vi "START6LED.vi"() -> ()   [LabVIEW 2024]
uses:
  <vilib>/Utility/file.llb/Read Delimited Spreadsheet (DBL).vi
panel:
  in  "Flow Rate Lower Limit 2":dbl
  in  "Flow Rate Upper Limit 2":dbl
  in  "Desired Flow Rate 3":dbl format="%_2f"
  in  "Initial RPM  3":dbl format="%_4f"
  in  "stop 2":bool
  out "Boolean":bool
  out "Waveform Chart 3":dbl[](graph)
  out "Waveform Chart 2":dbl[](graph)
  out "Flow Rate":dbl[](graph)
  in  "Color Box":u32(colorbox)
  # "Blood Flow Rate"
  # "Initial LVAD Speed (RPM)"
  # "Desired Flow Rate (L/min)"
  # "LVAD Speed"
  # "Upper Flow Rate Limit (L/min)"
  # "Lower Flow Rate Limit (L/min)"
  # "Optimal Flow State"
  # "Right Heart Waveform"
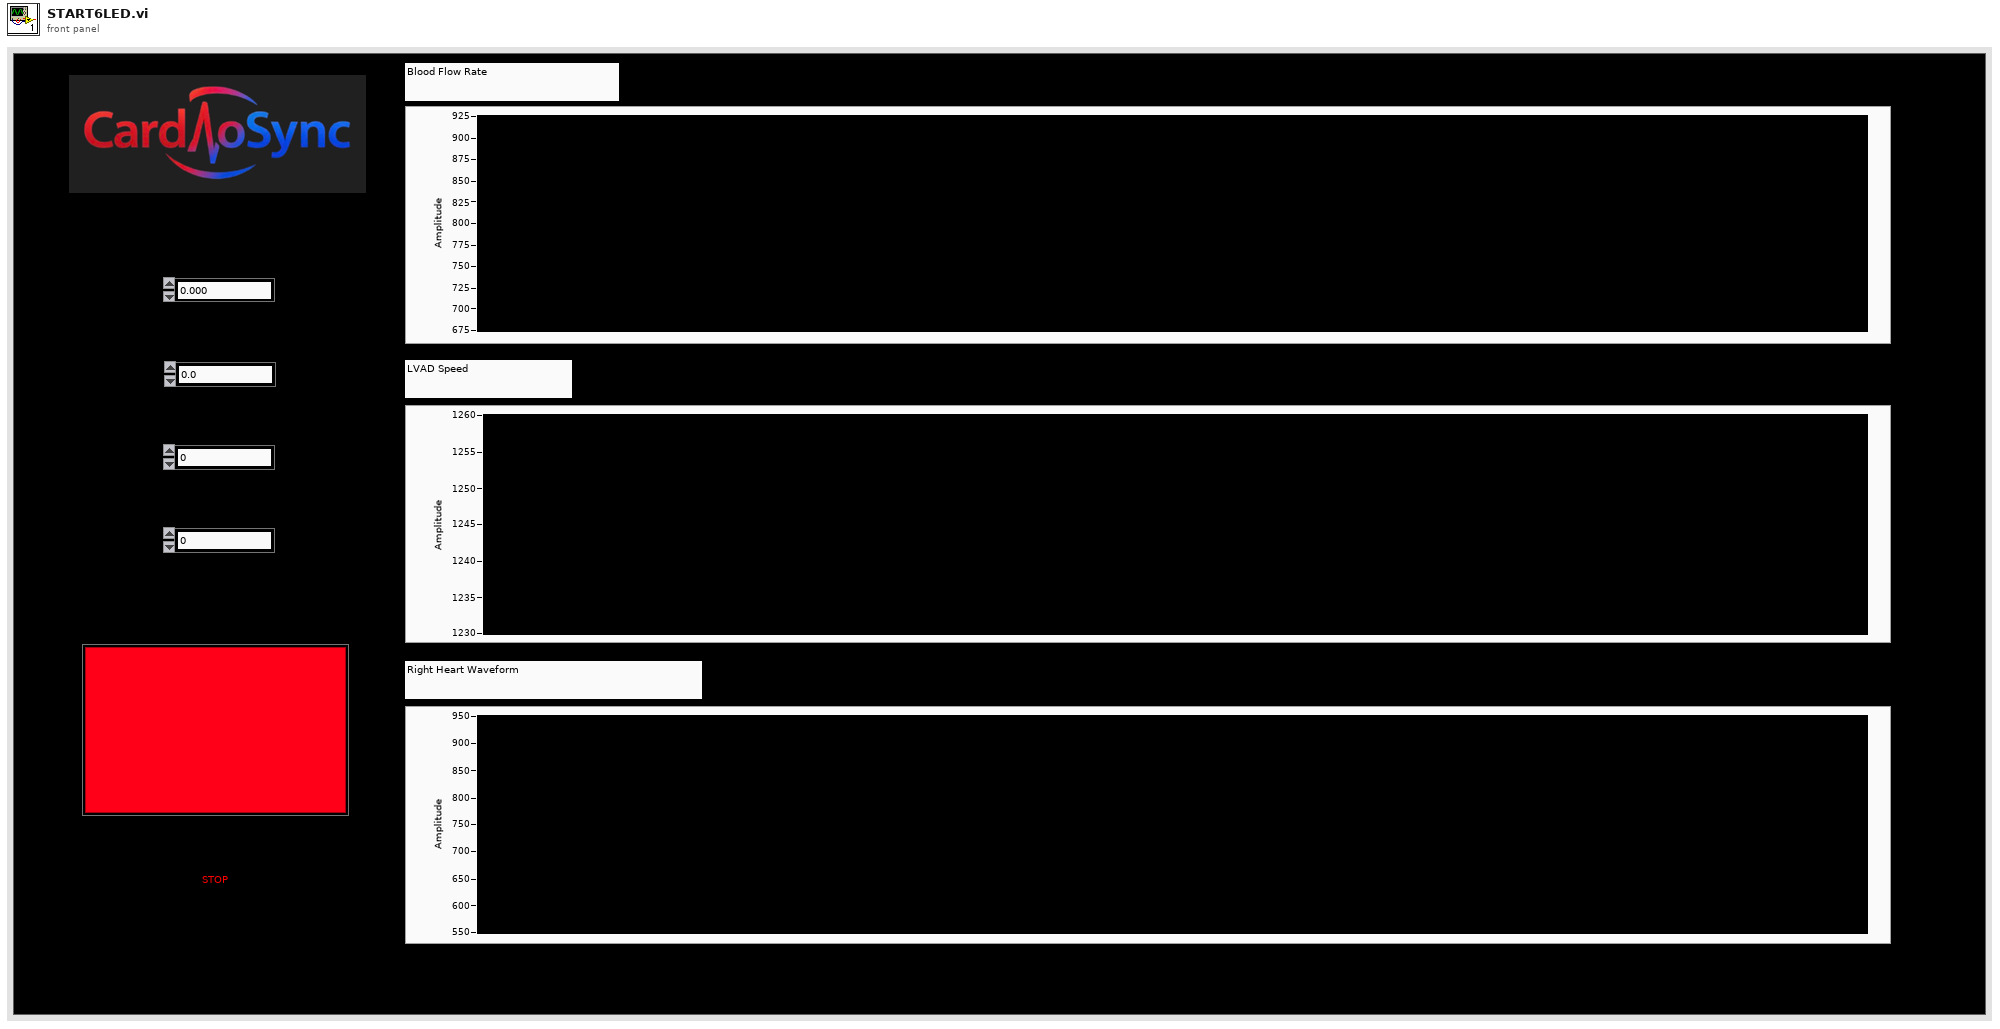
[diagram p1: front panel]
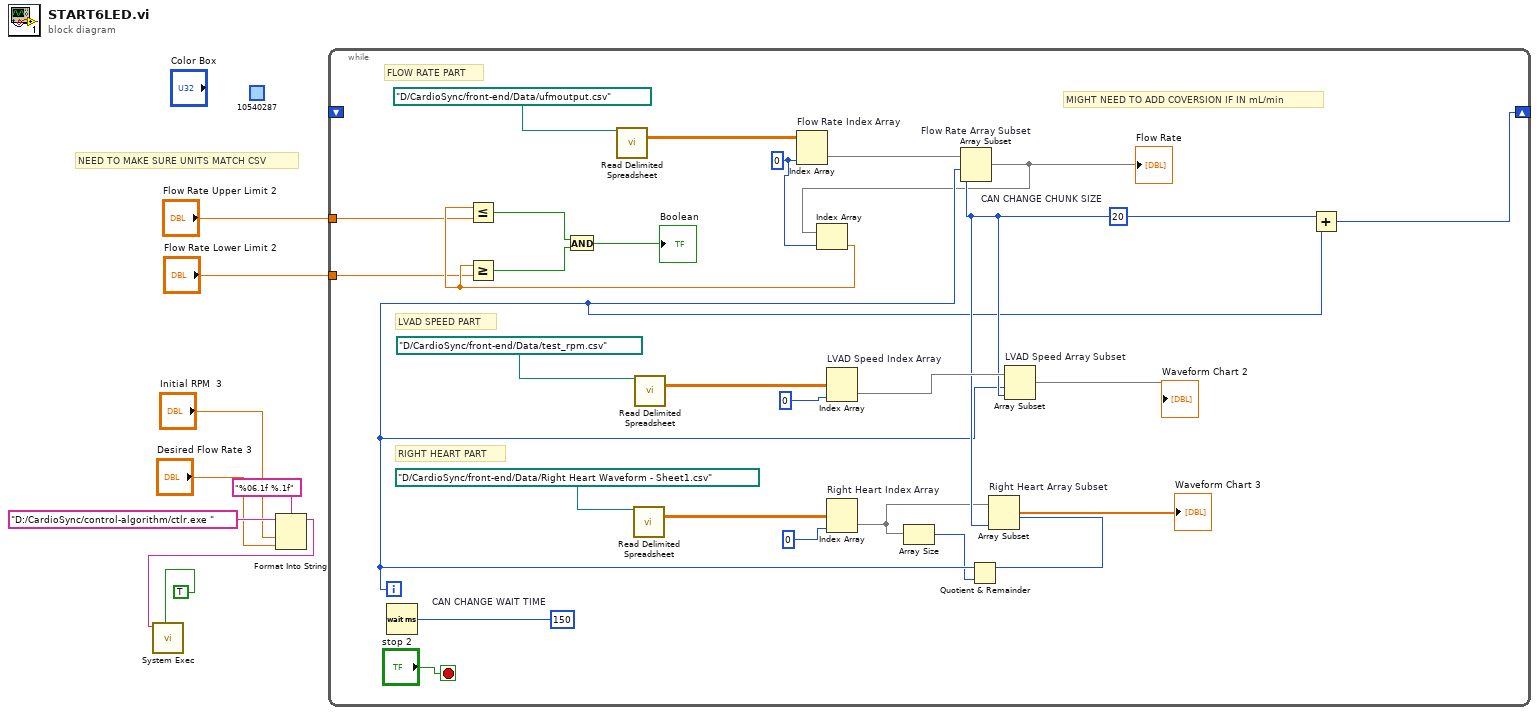
[diagram p0: block diagram]
diagram:
  (unwired) u32 10540287 ("Color Box 2")
  # "NEED TO MAKE SURE UNITS MATCH CSV"
  n1 = Format Into String(format string="%06.1f %.1f", initial string="D:/CardioSync/control-algorithm/ctlr.exe ", "Initial RPM  3", "Desired Flow Rate 3") -> (resulting string=w2:string)  [unwired: 1 in, 1 out]
  n2 = call <vilib>:"System Exec.vi"("wait until completion? (T)"=TRUE, "command line"=w2) -> ()  [unwired: 6 in, 4 out]
  n3 = while {
    shift-right: [w32] -> _
    shift-left: _ -> [_]
    tunnel: "Flow Rate Upper Limit 2" -> [w10]
    tunnel: "Flow Rate Lower Limit 2" -> [w9]
    i -> [w20]
    stop <- "stop 2" stop-if-true
    w33 = u32 150  # CAN CHANGE WAIT TIME
    w25 = 20  # CAN CHANGE CHUNK SIZE
    w13 = 0 ("disabled index (col)")
    # "MIGHT NEED TO ADD COVERSION IF IN mL/min"
    # "RIGHT HEART PART"
    # "LVAD SPEED PART"
    # "FLOW RATE PART"
    n4 = Wait (ms)(milliseconds to wait=w33) -> ()  [unwired: 1 out]
    n5 = call-poly <vilib>:"Read Delimited Spreadsheet.vi"("file path (dialog if empty)"=path "D:/CardioSync/front-end/Data/ufmoutput.csv") -> ("all rows"=w35:dbl[][])  [unwired: 9 in, 5 out]
    n6 = call-poly <vilib>:"Read Delimited Spreadsheet.vi"("file path (dialog if empty)"=path "D:/CardioSync/front-end/Data/Right Heart Waveform - Sheet1.csv") -> ("all rows"=w26:dbl[][])  [unwired: 9 in, 5 out]
    n7 = call-poly <vilib>:"Read Delimited Spreadsheet.vi"("file path (dialog if empty)"=path "D:/CardioSync/front-end/Data/test_rpm.csv") -> ("all rows"=w29:dbl[][])  [unwired: 9 in, 5 out]
    n8 = Index Array "Flow Rate Index Array"(array=w35, index (col)=w13) -> (element=w34:dbl[])  [unwired: 1 in]
    n9 = Index Array "LVAD Speed Index Array"(array=w29, index (col)=0 ("disabled index (col)")) -> (element=w28:dbl[])  [unwired: 1 in]
    n10 = Index Array "Right Heart Index Array"(array=w26, index (col)=0 ("disabled index (col)")) -> (element=w21:dbl[])  [unwired: 1 in]
    n11 = Array Size(array=w21) -> (size(s)=w19:i32)
    n12 = Array Subset "Flow Rate Array Subset"(array=w34, index=w20, length=w25) -> (w14:dbl[])
    "Flow Rate" <- w14
    n13 = Index Array(array=w14, index=w13) -> (element=w12:dbl)
    n14 = Less Or Equal?(x=w12, y=w10) -> (x <= y?=w17:bool)
    n15 = Greater Or Equal?(x=w12, y=w9) -> (x >= y?=w16:bool)
    n16 = And(x=w17, y=w16) -> (x .and. y?=→"Boolean":bool)
    n17 = Quotient & Remainder(x=w20, y=w19) -> (x-y*floor(x/y)=w18:i32)  [unwired: 1 out]
    n18 = Array Subset "Right Heart Array Subset"(array=w21, index=w18, length=w25) -> (→"Waveform Chart 3":dbl[])
    n19 = Array Subset "LVAD Speed Array Subset"(array=w28, index=w20, length=w25) -> (→"Waveform Chart 2":dbl[])
    n20 = Add(x=w25, y=w20) -> (x+y=w32:i32)
  }
